vi "Main (DAQ, 3 Tasks, Tag, Stream).vi"() -> ()   [LabVIEW 2018]
doc: "Datenerfassung - Producer/Consumer mit Zustandsmaschine und Tag Channel\n\n* Analoges Eingangssigna, Definition des\nDAQmx Kanals im NI Max\n* Realisierung mit eine Zustandsmaschine\n* Drei Schleifen (Tasks): Zustandsmaschine und Datenerfassung und Auswertung\n*Realisierung des User Interfaces mit Event Structure\n* Kommunikation benutzereingaben (Zustandsmaschine) zu Datenerfassung mit \"Tag Channel\" und \"Stream Channel\"\n* Anzeige der Events\n* Anzeige der Zustände \"Messung/Warten/Auswertung\""
uses:
  Type Definitions/States UI.ctl
  <vilib>/DAQmx/read.llb/DAQmx Read (Analog Wfm 1Chan NSamp).vi
  <extravilib>/ChannelInstances/Stream-wfm(dbl)/EndpointRead.vi
  <extravilib>/ChannelInstances/Stream-wfm(dbl)/Endpoint.vi
  <extravilib>/ChannelInstances/Tag-bool/Instantiate.vi
  <extravilib>/ChannelInstances/Tag-bool/Endpoint.vi
  <extravilib>/ChannelInstances/Stream-wfm(dbl)/Instantiate.vi
  <extravilib>/ChannelInstances/Stream-wfm(dbl)/)Channel.vi
  <resource>/ChannelSupport/_ChannelSupport/WaitIfNeeded.vi
  <vilib>/Waveform/WDTOps.llb/WDT Append Waveforms DBL.vi
  <extravilib>/ChannelInstances/Tag-bool/EndpointRead.vi
  <vilib>/DAQmx/miscellaneous.llb/DAQmx Fill In Error Info.vi
  <extravilib>/ChannelInstances/Tag-bool.lvlib
  <extravilib>/ChannelInstances/Stream-wfm(dbl).lvlib
panel:
  in  "Tab Control":enum32{"Graph", "Chart"}(tab)=enum."Chart"
  out "element":waveform(dbl)(graph)
  out "Waveform Chart":waveform(dbl)(graph)
  out "Messung":bool
  out "Events":string="Exit= 1"
  in  "Messung":bool
  in  "Exit":bool
  out "Anzeige":dbl(knob) scale=0.0..10.0 scale format="%1.1f"
  # "Datenerfassung - Producer/Consumer mit Zustandsmaschine und Tag sowie Stream Channel\n\n* Analoges Eingangssignal, Definition des\nDAQmx Kanals im NI Max\n*  Realisierung mit eine Zustandsmaschine\n* Zustandsmaschine nur für UI Events\n* Drei Schleifen (Tasks): Zustandsmaschine, Datenerfassung und Auswertung\n* Realisierung des User Interfaces mit Event Structure\n* Kommunikation Benutzereingaben (Zustandsmaschine) zu Datenerfassung mit \"Tag Channel\"\n* Daten per Stream Channel zum Zustand \"Auswertung\"\n* Anzeige der Events\n* Anzeige der Zustände \"Messung/Warten/Auswertung\"\n\nTiming\n* Task 1Khz Sampling Rate und 100 Samples\n* Gemessen jede 1sec (Timed loop)"
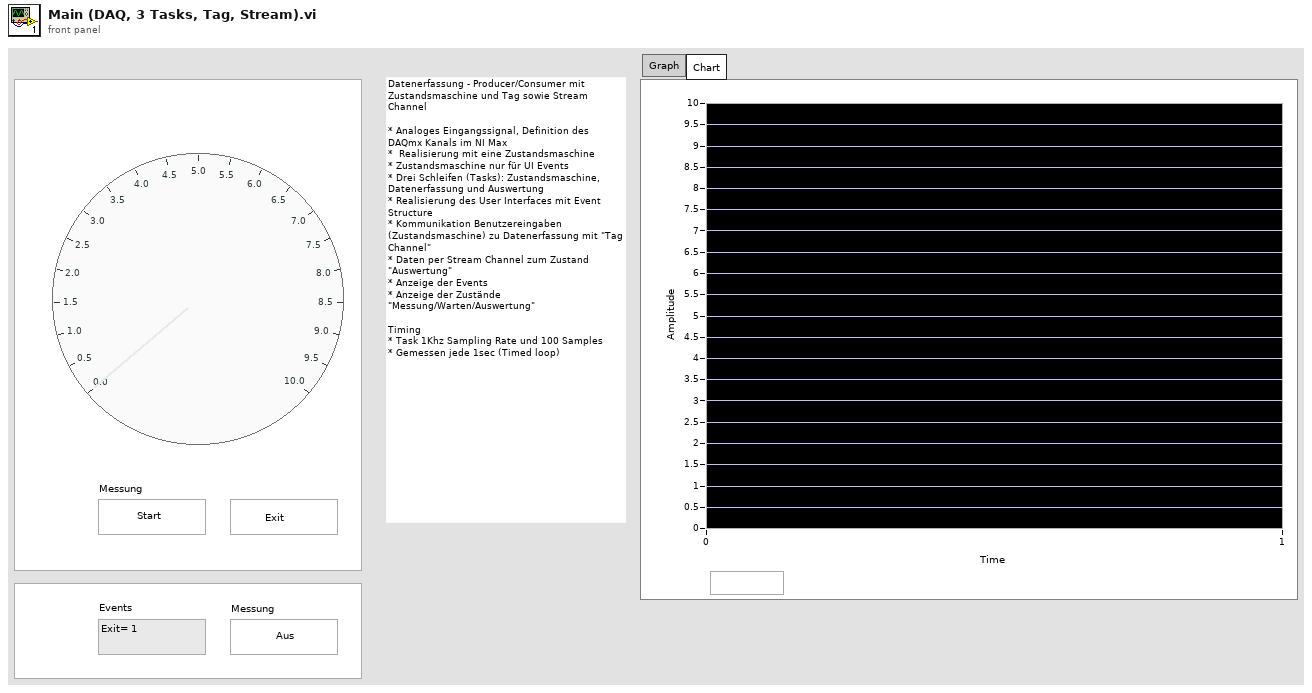
[diagram p1: front panel]
types:
  T1 = typedef "States UI.ctl" = enum16{"Initialize", "Wait for Event", "Exit"}
  T2 = typedef "Tag-bool.lvlib/))Channel.ctl" = refnum<queue>
  T3 = typedef "Stream-wfm(dbl).lvlib/)Channel.ctl" = refnum<queue>
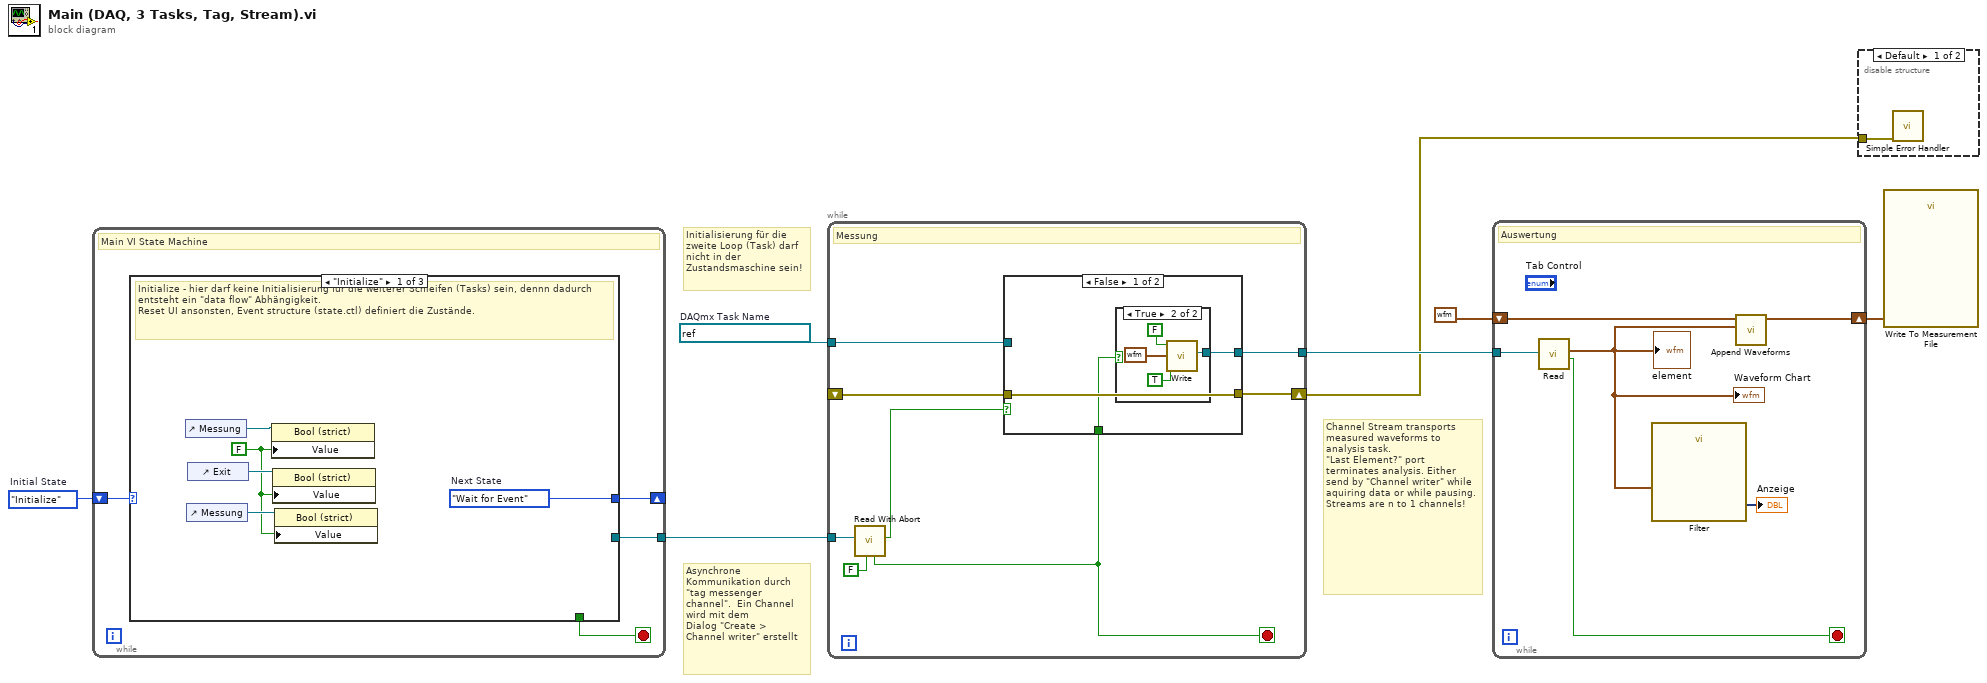
[diagram p0: block diagram]
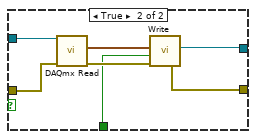
[diagram p3: hidden frame]
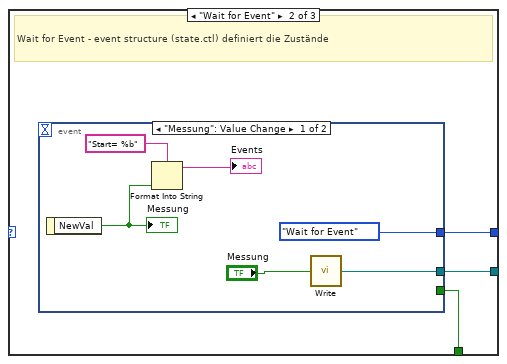
[diagram p4: hidden frame]
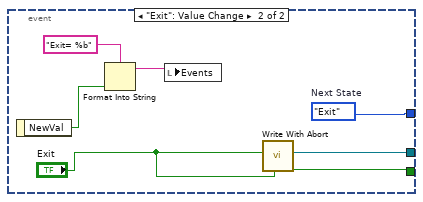
[diagram p5: hidden frame]
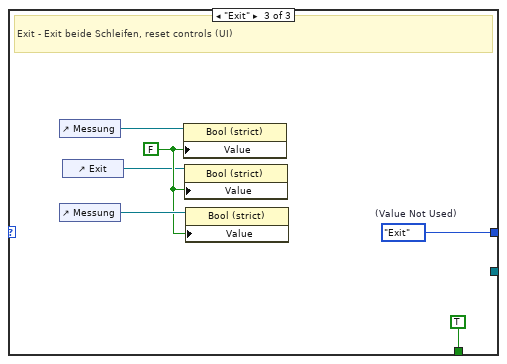
[diagram p6: hidden frame]
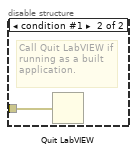
[diagram p7: hidden frame]
diagram:
  w5 = refnum<k21> "Spannung_1kHz100"  # DAQmx Task Name
  w7 = States_UI."Initialize"  # Initial State
  # "Channel Stream transports\nmeasured waveforms to analysis task.\n\"Last Element?\" port terminates analysis. Either send by \"Channel writer\" while aquiring data or while pausing. Streams are n to 1 channels!"
  # "Initialisierung für die zweite Loop (Task) darf\nnicht in der Zustandsmaschine sein!"
  # "Asynchrone Kommunikation durch\n\"tag messenger channel\".  Ein Channel wird mit dem\nDialog \"Create > Channel writer\" erstellt"
  n1 = while {
    shift-right: [w10] -> _
    shift-left: w7 -> [w11]
    tunnel: [w8] -> w1
    stop <- w9 stop-if-true
    # "Main VI State Machine"
    n2 = case shown="\"Initialize\"" w11 {
      tunnel: [w16 w19 w38] -> w10
      tunnel: [_ w17 TRUE ("Stop Loop?")] -> w9
      tunnel: [_ w18 _] -> w8
      frame "Initialize" {
        w12 = FALSE ("Value")
        w16 = States_UI."Wait for Event"  # Next State
        # "Initialize - hier darf keine Initialisierung für die weiterer Schleifen (Tasks) sein, dennn dadurch entsteht ein \"data flow\" Abhängigkeit. \nReset UI ansonsten, Event structure (state.ctl) definiert die Zustände."
        n3 = control-ref of="Messung"() -> (w15:refnum<vi>)
        n4 = control-ref of="Messung"() -> (w13:refnum<vi>)
        n5 = control-ref of="Exit"() -> (w14:refnum<vi>)
        n6 = property class="Bool (strict)"(reference=w15, "Value"=w12) -> ()  [unwired: 1 in, 2 out]
        n7 = property class="Bool (strict)"(reference=w14, "Value"=w12) -> ()  [unwired: 1 in, 2 out]
        n8 = property class="Bool (strict)"(reference=w13, "Value"=w12) -> ()  [unwired: 1 in, 2 out]
      }
      frame "Wait for Event" {
        # "Wait for Event - event structure (state.ctl) definiert die Zustände"
        n9 = event shown="[0] \"Messung\": Value Change" {
          selector: _ -> [_ _]
          dyn-events: _ -> [_ _]
          timeout: _ -> [_ _]
          tunnel: [States_UI."Wait for Event" ("Next State") w32] -> w19
          tunnel: [w20 w28] -> w18
          tunnel: [_ w26] -> w17
          event "Messung": Value Change {
            n10 = event-data() -> ("NewVal"=w22:bool)  [unwired: 1 in]
            "Messung" <- w22
            n11 = Format Into String(format string="Start= %b", w22) -> (resulting string=→"Events":string)  [unwired: 2 in, 1 out]
            n12 = call <extravilib>:"Write.vi"("element"="Messung") -> ("channel"=w20:T2)  [unwired: 1 out]
          }
          event "Exit": Value Change {
            w32 = States_UI."Exit"  # Next State
            n13 = event-data() -> ("NewVal"=w30:bool)  [unwired: 1 in]
            n14 = Format Into String(format string="Exit= %b", w30) -> (resulting string=w31:string)  [unwired: 2 in, 1 out]
            n15 = local write "Events"(w31) -> ()
            n16 = call <extravilib>:"Write With Abort.vi"("abort"="Exit", "element"="Exit") -> ("channel"=w28:T2, "aborted?"=w26:bool)  [unwired: 7 in, 1 out]
          }
        }
      }
      frame "Exit" {
        w35 = FALSE ("Value")
        w38 = States_UI."Exit"  # (Value Not Used)
        # "Exit - Exit beide Schleifen, reset controls (UI)"
        n17 = control-ref of="Messung"() -> (w37:refnum<vi>)
        n18 = control-ref of="Messung"() -> (w36:refnum<vi>)
        n19 = control-ref of="Exit"() -> (w34:refnum<vi>)
        n20 = property class="Bool (strict)"(reference=w37, "Value"=w35) -> ()  [unwired: 1 in, 2 out]
        n21 = property class="Bool (strict)"(reference=w34, "Value"=w35) -> ()  [unwired: 1 in, 2 out]
        n22 = property class="Bool (strict)"(reference=w36, "Value"=w35) -> ()  [unwired: 1 in, 2 out]
      }
    }
  }
  n23 = while {
    shift-right: [w46] -> w4
    shift-left: _ -> [w45]
    tunnel: [w40] -> w6
    tunnel: w5 -> [w44]
    tunnel: w1 -> [w43]
    stop <- w39 stop-if-true
    # "Messung"
    n24 = call <extravilib>:"Read With Abort.vi"("abort"=FALSE, "channel"=w43) -> ("element"=w42:bool, "aborted?"=w39:bool)  [unwired: 7 in, 1 out]
    n25 = case shown="False" w42 {
      tunnel: [w49 w59] -> w46
      tunnel: w45 -> [w49 w58]
      tunnel: w44 -> [_ w57]
      tunnel: w39 -> [w47 w55]
      tunnel: [w48 w54] -> w40
      frame False {
        n26 = case shown="True" w47 {
          tunnel: [_ w53] -> w48
          frame False {
          }
          frame True {
            n27 = call <extravilib>:"Write.vi"("last element? (F)"=TRUE, "element"=waveform(dbl) {"t0"=timestamp(0 s since 1904-01-01), "dt"=1.0, "Y"=[]}, "element valid? (T)"=FALSE) -> ("channel"=w53:T3)  [unwired: 6 in, 2 out]
          }
        }
      }
      frame True {
        n28 = call-poly <vilib>:"DAQmx Read.vi"("task/channels in"=w57, "error in"=w58) -> ("data"=w56:waveform(dbl), "error out"=w59:errorcluster)  [unwired: 11 in, 1 out]
        n29 = call <extravilib>:"Write.vi"("last element? (F)"=w55, "element"=w56) -> ("channel"=w54:T3)  [unwired: 7 in, 2 out]
      }
    }
  }
  n30 = while {
    tunnel: w6 -> [w65]
    shift-right: [w62] -> w2
    shift-left: waveform(dbl) {"t0"=timestamp(0 s since 1904-01-01), "dt"=1.0, "Y"=[]} ("Waveform") -> [w63]
    stop <- w60 stop-if-true
    # "Auswertung"
    n31 = call <extravilib>:"Read.vi"("channel"=w65) -> ("last element?"=w60:bool, "element"=w64:waveform(dbl))  [unwired: 6 in, 3 out]
    "element" <- w64
    "Waveform Chart" <- w64
    n32 = call "Filter"("Signal"=w64) -> ("Filtered Signal"=→"Anzeige":dynamicdata)  [unwired: 9 in, 1 out]
    n33 = call-poly <vilib>:"Append Waveforms.vi"("waveform B"=w64, "waveform A"=w63) -> ("waveform out"=w62:waveform(dbl))  [unwired: 8 in, 1 out]
  }
  n34 = disable-structure shown="Default" {
    disable-tunnel: w4 -> [w66 w67]
    frame condition #0 (active) {
      n35 = call <vilib>:"Simple Error Handler.vi"("error in (no error)"=w66) -> ()  [unwired: 4 in, 5 out]
    }
    frame condition #1 {
      # "Call Quit LabVIEW if running as a built application."
      n36 = Quit LabVIEW(quit? (T)=w67) -> ()
    }
  }
  n37 = call "Write To Measurement File"("Signals"=w2) -> ()  [unwired: 16 in, 3 out]
